vi "Write Tags.vi"(8 "error in (no error)":errorcluster, 11 "State in":T1={"State"=enum."Idle", "Start Time"=timestamp(0 s since 1904-01-01), "Configuration"={"Cycle Period"=0.0, "Bronkhorst M13"={"VISA resource name"="", "Simulated?"=FALSE}, "Flow Meter Type"="", "Bronkhorst M14"={"VISA resource name"="", "Simulated?"=FALSE}}, "Current Time"=timestamp(0 s since 1904-01-01), "First Iteration"=FALSE, "Data"={"Flow Meter Read(g/min)"=0.0, "Density"=0.0, "Temp (C)"=0.0}, "Process Name"="", "Log Started"=FALSE}) -> (0 "error out":errorcluster, 3 "State out":T1={"State"=enum."Idle", "Start Time"=timestamp(0 s since 1904-01-01), "Configuration"={"Cycle Period"=0.0, "Bronkhorst M13"={"VISA resource name"="", "Simulated?"=FALSE}, "Flow Meter Type"="", "Bronkhorst M14"={"VISA resource name"="", "Simulated?"=FALSE}}, "Current Time"=timestamp(0 s since 1904-01-01), "First Iteration"=FALSE, "Data"={"Flow Meter Read(g/min)"=0.0, "Density"=0.0, "Temp (C)"=0.0}, "Process Name"="", "Log Started"=FALSE})   [LabVIEW 2018, in "Flow Module.lvlib" / "Flow Module Engine.lvlib"]
uses:
  Flow Module Engine.lvlib
  State Cluster.ctl
  State Enum.ctl
  Feed Module/Controls/Flow Module Settings Cluster.ctl
  Mettler Toledo/Controls/Settings Cluster.ctl
  Tag VIs/Tag FGV Operation Enum.ctl
  Shared Variables/Dynamic Shared Variables.lvlib
  Flow Module.lvlib
  Mettler Toledo/Mettler Toledo.lvlib
panel:
  # "Flow Meter Settings"
  # "Flow Meter Settings"
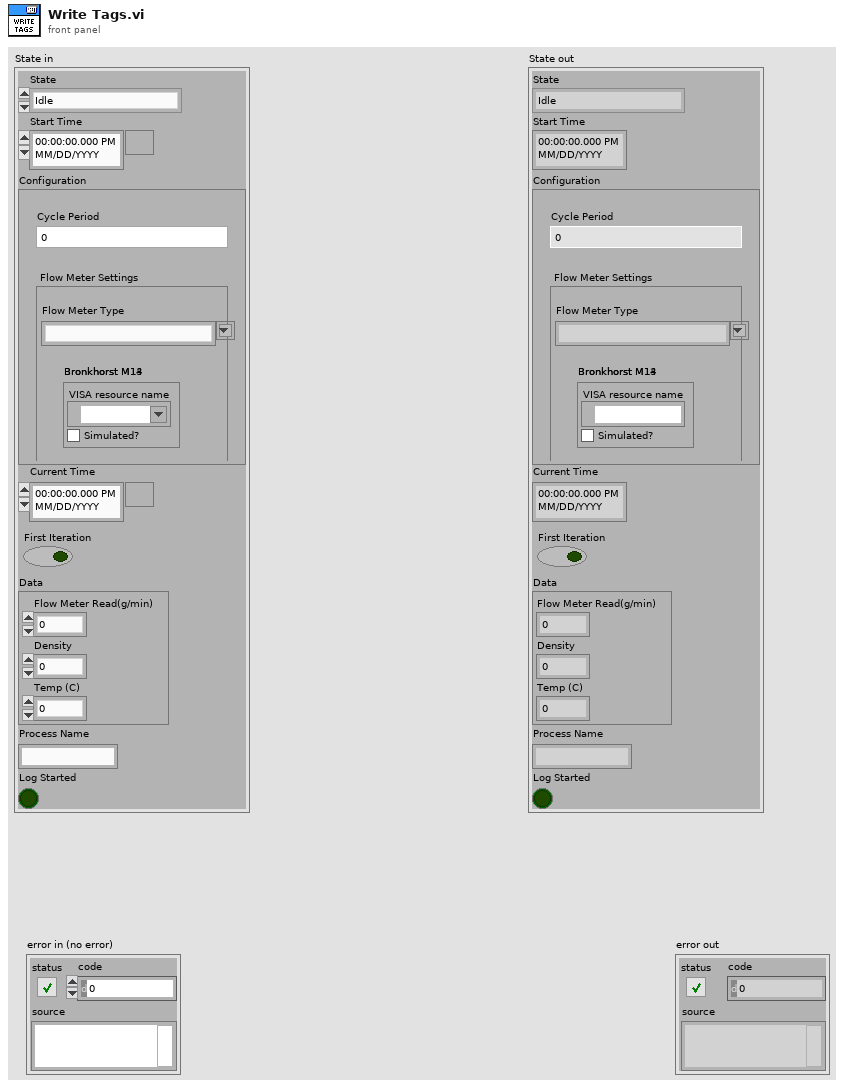
[diagram p1: front panel]
types:
  T1 = typedef "Flow Module.lvlib/Flow Module Engine.lvlib/State Cluster.ctl" = cluster{"State":T2, "Start Time":timestamp, "Configuration":T3, "Current Time":timestamp, "First Iteration":bool, "Data":cluster{"Flow Meter Read(g/min)":dbl, "Density":dbl, "Temp (C)":dbl}, "Process Name":string, "Log Started":bool}
  T2 = typedef "Flow Module.lvlib/Flow Module Engine.lvlib/State Enum.ctl" = enum16{"Measuring", "Idle"}
  T3 = typedef "Flow Module.lvlib/Flow Module Settings Cluster.ctl" = cluster{"Cycle Period":dbl, "Bronkhorst M13":T4, "Flow Meter Type":string, "Bronkhorst M14":T4}
  T4 = typedef "Mettler Toledo.lvlib/Settings Cluster.ctl" = cluster{"VISA resource name":refnum<visa-resource-name>, "Simulated?":bool}
  T5 = typedef "Tag FGV Operation Enum.ctl" = enum16{"Init", "Set Notification Queue", "Create Tag", "Commit", "Write Tag (Numeric)", "Write Tag (Boolean)", "Read All Tags", "Read One Tag", "Delete Tag Category", "Set Alarm Parameters (Numeric)", "Set Alarm Parameters (Boolean)", "Enable All Alarms", "Disable All Alarms", "Delete All Tags", "Read Alarms", "Ack Alarm", "Read Alarm Parameters (Numeric)", "Read Alarm Parameters (Boolean)"}
  T6 = typedef "Flow Module.lvlib/Tag Cluster.ctl" = cluster{"Flow Tag":string, "Input Disconnected":string, "Density Tag":string, "Temp Tag":string}
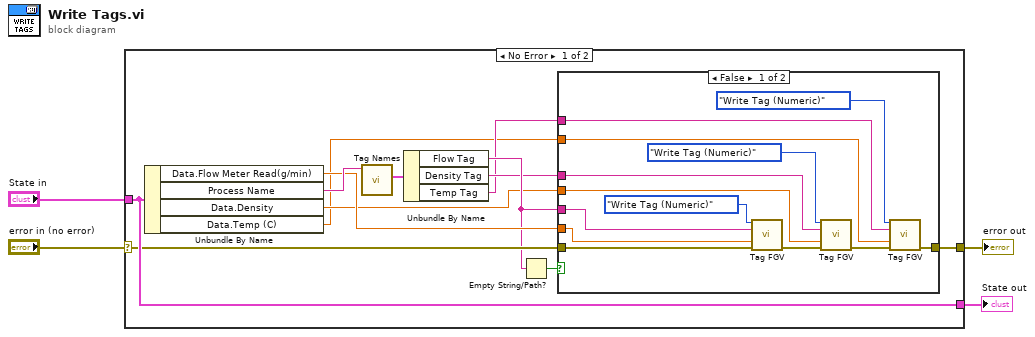
[diagram p0: block diagram]
diagram:
  n1 = case shown="No Error" "error in (no error)" {
    selector: "error in (no error)" -> [w12 w32]
    tunnel: [w15 w32] -> w3
    tunnel: "State in" -> [w13 w31]
    tunnel: [w13 w31] -> w1
    frame No Error {
      n2 = Unbundle By Name(w13) -> ("Data.Flow Meter Read(g/min)"=w11:dbl, "Process Name"=w16:string, "Data.Density"=w7:dbl, "Data.Temp (C)"=w5:dbl)
      n3 = call "Tag Names.vi"("Process Name"=w16) -> ("Flow Tags"=w10:T6)  [unwired: 8 in, 2 out]
      n4 = Unbundle By Name(w10) -> ("Flow Tag"=w9:string, "Density Tag"=w8:string, "Temp Tag"=w6:string)
      n5 = Empty String/Path?(string/path=w9) -> (empty?=w14:bool)
      n6 = case shown="False" w14 {
        tunnel: [w19 w30] -> w15
        tunnel: w12 -> [w28 w30]
        tunnel: w11 -> [w27 _]
        tunnel: w9 -> [w26 _]
        tunnel: w8 -> [w23 _]
        tunnel: w7 -> [w22 _]
        tunnel: w6 -> [w18 _]
        tunnel: w5 -> [w17 _]
        frame False {
          n7 = call "Tag FGV.vi"("Operation"=Tag_FGV_Operation_Enum."Write Tag (Numeric)", "Tag Name"=w26, "Data"=w27, "error in (no error)"=w28) -> ("error out"=w24:errorcluster)  [unwired: 4 in, 7 out]
          n8 = call "Tag FGV.vi"("Operation"=Tag_FGV_Operation_Enum."Write Tag (Numeric)", "Tag Name"=w23, "Data"=w22, "error in (no error)"=w24) -> ("error out"=w20:errorcluster)  [unwired: 4 in, 7 out]
          n9 = call "Tag FGV.vi"("Operation"=Tag_FGV_Operation_Enum."Write Tag (Numeric)", "Tag Name"=w18, "Data"=w17, "error in (no error)"=w20) -> ("error out"=w19:errorcluster)  [unwired: 4 in, 7 out]
        }
        frame True {
        }
      }
    }
    frame Error {
    }
  }
  "error out" <- w3
  "State out" <- w1
